vi "Configure Peak Search.vi"(0 "VISA resource name":refnum<visa-resource-name>, 5 "Marker (0:Marker 1)":i32(ring) items=["Marker 1", "Marker 2", "Marker 3", "Marker 4", "Marker 5", "Marker 6", "Marker 7", "Marker 8", "Marker 9", "Marker 10"], 7 "Search Mode (0:Peak Search)":i32(ring) items=["Peak Search", "Next Peak", "Minimum Search", "Next Minimum", "Parameter Set", "Power Peak Search", "Power Next Peak", "Power Minimum Search", "Power Next Minimum", "Power Parameter Set"], 9 "Search Threshold (0:Off)":i32(ring) items=["Off", "On", "Above", "Below"], 11 "error in (no error)":errorcluster, 12 "Threshold Level (-90.00dBm)":dbl=-90.0 min=-150.0 max=50.0 format="%.2f", 13 "Resolution (0.001dB)":dbl=0.001 min=0.001 max=100.0 format="%.3f") -> (4 "VISA resource name out":refnum<visa-resource-name>, 15 "error out":errorcluster)   [LabVIEW 2020, in "Anritsu Signal Analyzer Series.lvlib"]
doc: "Configures the Peak and Power Search settings of the spectrum analyzer."
uses:
  Anritsu Signal Analyzer Series.lvlib
panel:
  # "dBm"
  # "dB"
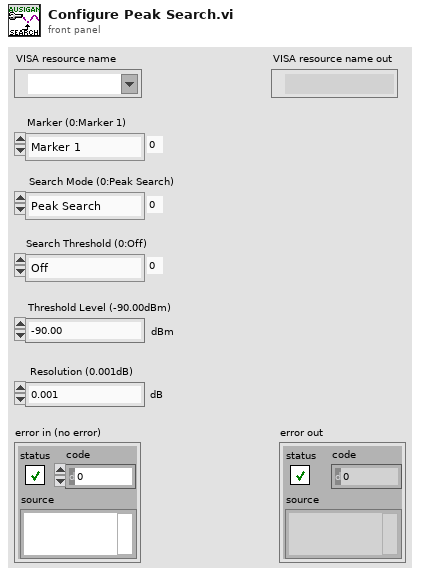
[diagram p1: front panel]
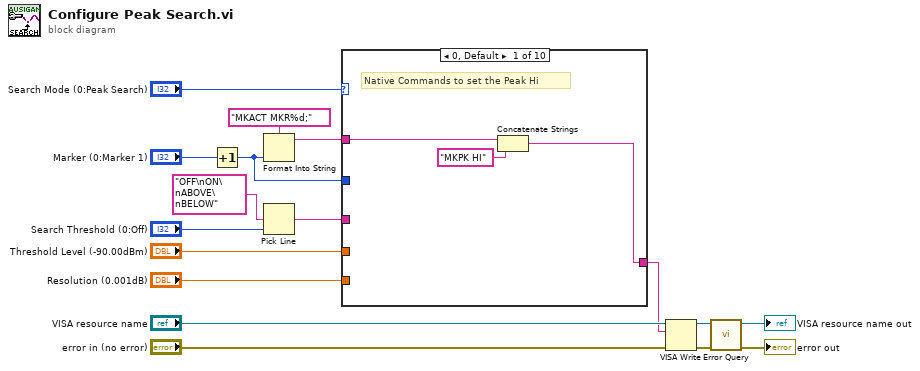
[diagram p0: block diagram]
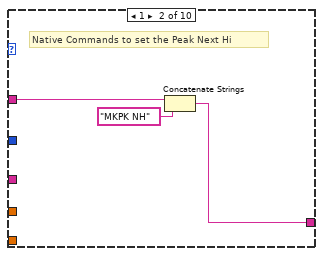
[diagram p2: hidden frame]
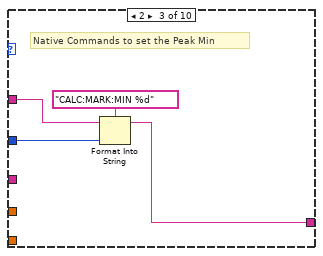
[diagram p3: hidden frame]
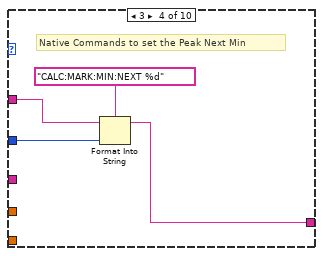
[diagram p4: hidden frame]
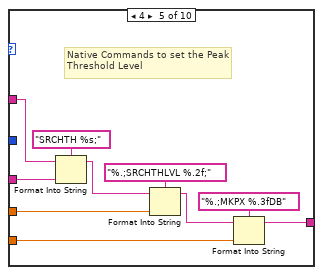
[diagram p5: hidden frame]
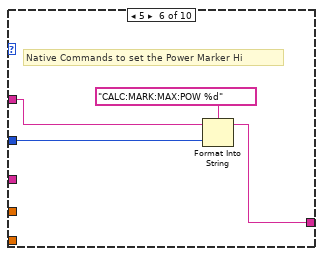
[diagram p6: hidden frame]
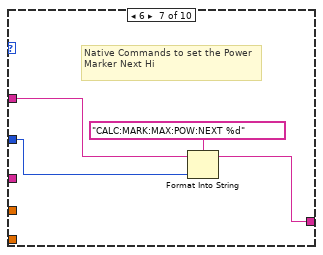
[diagram p7: hidden frame]
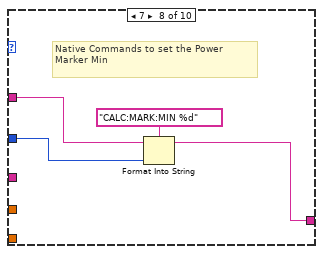
[diagram p8: hidden frame]
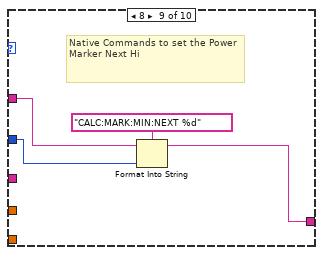
[diagram p9: hidden frame]
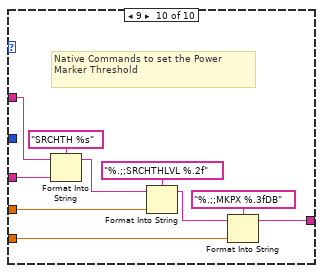
[diagram p10: hidden frame]
diagram:
  n1 = Increment(x="Marker (0:Marker 1)") -> (x+1=w1:i32)
  n2 = Format Into String(format string="MKACT MKR%d;" ("_CommandSet"), w1) -> (resulting string=w2:string)  [unwired: 2 in, 1 out]
  n3 = Pick Line(multi-line string="OFF\nON\nABOVE\nBELOW" ("複数行文字列"), line index="Search Threshold (0:Off)") -> (output string=w3:string)  [unwired: 1 in]
  n4 = case shown="0, Default" "Search Mode (0:Peak Search)" {
    tunnel: w2 -> [w20 w23 w26 w30 w40 w44 w48 w52 w56 w62]
    tunnel: w1 -> [_ _ w24 w28 _ w43 w47 w51 w55 _]
    tunnel: w3 -> [_ _ _ _ w41 _ _ _ _ w58]
    tunnel: "Threshold Level (-90.00dBm)" -> [_ _ _ _ w36 _ _ _ _ w61]
    tunnel: "Resolution (0.001dB)" -> [_ _ _ _ w33 _ _ _ _ w60]
    tunnel: [w18 w21 w25 w29 w32 w42 w46 w50 w54 w59] -> w6
    frame 0, Default {
      # "Native Commands to set the Peak Hi"
      n5 = Concatenate Strings(w20, "MKPK HI" ("_CommandSet")) -> (w18:string)
    }
    frame 1 {
      # "Native Commands to set the Peak Next Hi"
      n6 = Concatenate Strings(w23, "MKPK NH" ("_CommandSet")) -> (w21:string)
    }
    frame 2 {
      # "Native Commands to set the Peak Min"
      n7 = Format Into String(format string="CALC:MARK:MIN %d", initial string=w26, w24) -> (resulting string=w25:string)  [unwired: 1 in, 1 out]
    }
    frame 3 {
      # "Native Commands to set the Peak Next Min"
      n8 = Format Into String(format string="CALC:MARK:MIN:NEXT %d", initial string=w30, w28) -> (resulting string=w29:string)  [unwired: 1 in, 1 out]
    }
    frame 4 {
      # "Native Commands to set the Peak Threshold Level"
      n9 = Format Into String(format string="SRCHTH %s;" ("_CommandSet"), initial string=w40, w41) -> (resulting string=w37:string)  [unwired: 1 in, 1 out]
      n10 = Format Into String(format string="%.;SRCHTHLVL %.2f;" ("Format String"), initial string=w37, w36) -> (resulting string=w34:string)  [unwired: 1 in, 1 out]
      n11 = Format Into String(format string="%.;MKPX %.3fDB" ("Format String"), initial string=w34, w33) -> (resulting string=w32:string)  [unwired: 1 in, 1 out]
    }
    frame 5 {
      # "Native Commands to set the Power Marker Hi"
      n12 = Format Into String(format string="CALC:MARK:MAX:POW %d" ("_CommandSet"), initial string=w44, w43) -> (resulting string=w42:string)  [unwired: 1 in, 1 out]
    }
    frame 6 {
      # "Native Commands to set the Power Marker Next Hi"
      n13 = Format Into String(format string="CALC:MARK:MAX:POW:NEXT %d" ("_CommandSet"), initial string=w48, w47) -> (resulting string=w46:string)  [unwired: 1 in, 1 out]
    }
    frame 7 {
      # "Native Commands to set the Power Marker Min"
      n14 = Format Into String(format string="CALC:MARK:MIN %d" ("_CommandSet"), initial string=w52, w51) -> (resulting string=w50:string)  [unwired: 1 in, 1 out]
    }
    frame 8 {
      # "Native Commands to set the Power Marker Next Hi"
      n15 = Format Into String(format string="CALC:MARK:MIN:NEXT %d" ("_CommandSet"), initial string=w56, w55) -> (resulting string=w54:string)  [unwired: 1 in, 1 out]
    }
    frame 9 {
      # "Native Commands to set the Power Marker Threshold"
      n16 = Format Into String(format string="SRCHTH %s" ("_CommandSet"), initial string=w62, w58) -> (resulting string=w65:string)  [unwired: 1 in, 1 out]
      n17 = Format Into String(format string="%.;;SRCHTHLVL %.2f" ("Format String"), initial string=w65, w61) -> (resulting string=w64:string)  [unwired: 1 in, 1 out]
      n18 = Format Into String(format string="%.;;MKPX %.3fDB" ("Format String"), initial string=w64, w60) -> (resulting string=w59:string)  [unwired: 1 in, 1 out]
    }
  }
  n19 = VISA Write(VISA resource name="VISA resource name", write buffer=w6, error in (no error)="error in (no error)") -> (VISA resource name out=w7:refnum<visa-resource-name>, error out=w8:errorcluster)  [unwired: 1 out]
  n20 = call "Error Query.vi"("error in (no error)"=w8, "VISA resource name"=w7) -> ("error out"=→"error out":errorcluster, "VISA resource name out"=→"VISA resource name out":refnum<visa-resource-name>)  [unwired: 6 in, 2 out]
